vi "Get Method.vi"(8 "error in (no error)":errorcluster, 11 "Request in":refnum<class "Request.lvclass">) -> (0 "error out":errorcluster, 2 "Method":T1, 3 "Request out":refnum<class "Request.lvclass">)   [LabVIEW 2020, in "HTTP Utils.lvlib" / "Request.lvclass"]
uses:
  Request.lvclass
  Method.ctl
  Request.lvclass/Request.ctl
  HTTP Utils.lvlib
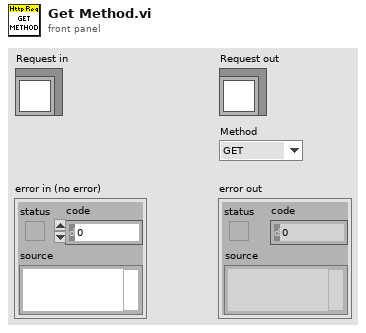
[diagram p1: front panel]
types:
  T1 = typedef "HTTP Utils.lvlib/Method.ctl" = enum16{"GET", "HEAD", "POST", "PUT", "DELETE", "CONNECT", "OPTIONS", "TRACE", "PATCH"}
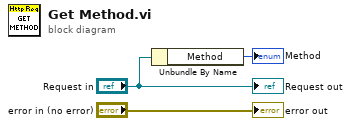
[diagram p0: block diagram]
diagram:
  n1 = Unbundle By Name("Request in") -> ("Method"=→"Method":T1)
  "error out" <- "error in (no error)"
  "Request out" <- "Request in"
